vi "Run Filter.vi"(8 "error in (no error)":errorcluster, 10 "resource entries in":T1[](array[typedef]) {"FPGA CD Ref" format="%.0x"; "reserver" format="%.0x"}, 11 "Input Type Filter in":refnum<class "Input Type Filter.lvclass">) -> (0 "error out":errorcluster, 2 "resource entries out":T1[](array[typedef]) {"FPGA CD Ref" format="%.0x"; "reserver" format="%.0x"})   [LabVIEW 2016, in "Input Type Filter.lvclass"]
uses:
  Input Type Filter.lvclass
  Server/viz_entry.ctl
  <vilib>/NI Veristand/Custom Device API/Custom Device Item Ref.ctl
  Input Type Filter.lvclass/Input Type Filter.ctl
  <vilib>/NI VeriStand/Custom Device API/Custom Device API.lvlib
  Server/RM.Server.lvlib
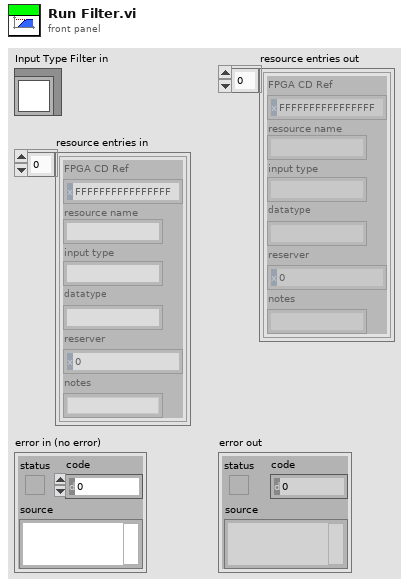
[diagram p1: front panel]
types:
  T1 = typedef "RM.Server.lvlib/viz_entry.ctl" = cluster{"FPGA CD Ref":T2, "resource name":string, "input type":string, "datatype":string, "reserver":T2, "notes":string}
  T2 = typedef "Custom Device API.lvlib/Custom Device Item Ref.ctl" = u64
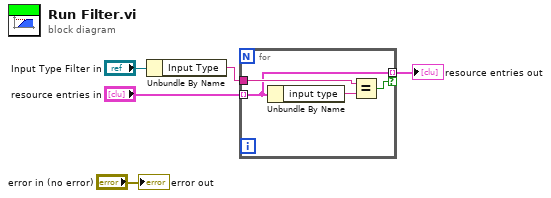
[diagram p0: block diagram]
diagram:
  n1 = Unbundle By Name("Input Type Filter in") -> ("Input Type"=w4:string)
  n2 = for {
    tunnel: w4 -> [w9]
    tunnel: "resource entries in" -> [w7] mode=indexing
    tunnel: [w7] -> w2 mode=indexing if=w6
    n3 = Unbundle By Name(w7) -> ("input type"=w8:string)
    n4 = Equal?(x=w9, y=w8) -> (x = y?=w6:bool)
  }
  "resource entries out" <- w2
  "error out" <- "error in (no error)"
